vi "Write Tasks names_.vi"(8 "error in (no error)":errorcluster, 10 "Tasks names":string[](array[string]), 11 "DAQmxTaksContainer_General in":refnum<class "DAQmxTaksContainer_General.lvclass">) -> (0 "error out":errorcluster, 3 "DAQmxTaksContainer_General out":refnum<class "DAQmxTaksContainer_General.lvclass">)   [LabVIEW 2015]
uses:
  DAQmxTaksContainer_General.lvclass
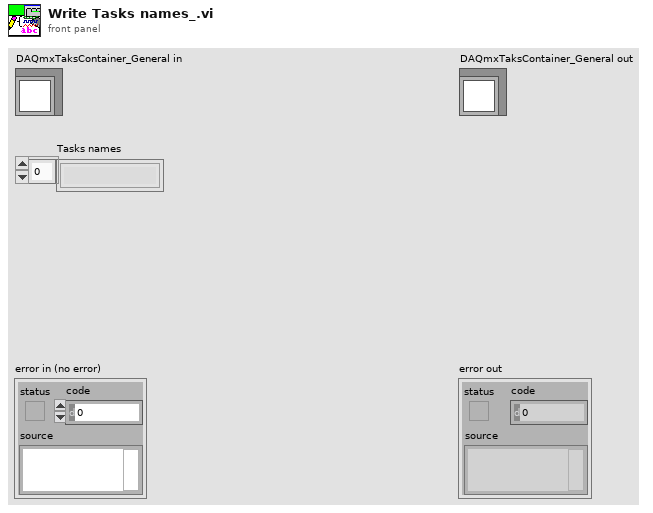
[diagram p1: front panel]
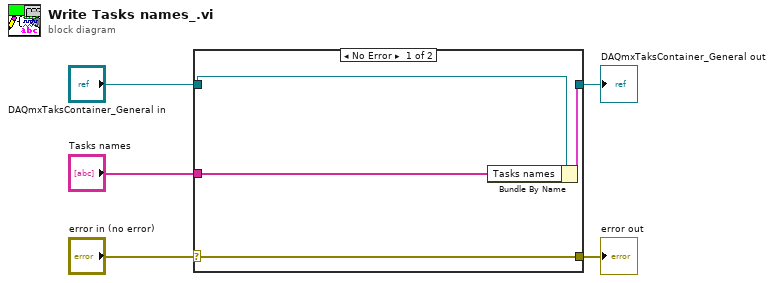
[diagram p0: block diagram]
diagram:
  n1 = case shown="No Error" "error in (no error)" {
    selector: "error in (no error)" -> [w9 w10]
    tunnel: [w9 w10] -> w4
    tunnel: [w7 w11] -> w2
    tunnel: "DAQmxTaksContainer_General in" -> [w8 w11]
    tunnel: "Tasks names" -> [w6 _]
    frame No Error {
      n2 = Bundle By Name(cluster=w8, "Tasks names"=w6) -> (w7:cluster{})
    }
    frame Error {
    }
  }
  "error out" <- w4
  "DAQmxTaksContainer_General out" <- w2
